vi "Get Sensor Objects Signals.vi"(7 "Filter Cluster":string="RDB_SENSOR_STATE", 8 "error in (no error)":errorcluster) -> (0 "error out (no error)":errorcluster, 1 "Sensor Signals":string[](array[string]), 2 "Sensor Names":string[](array[string]))   [LabVIEW 2023, in "Vires VTD System Explorer.lvlib"]
uses:
  Vires VTD System Explorer.lvlib
  <vilib>/xnet/xnet.llb/XNET String To IO Name (Database Alias).vi
  <resource>/objmgr/xnet.rc
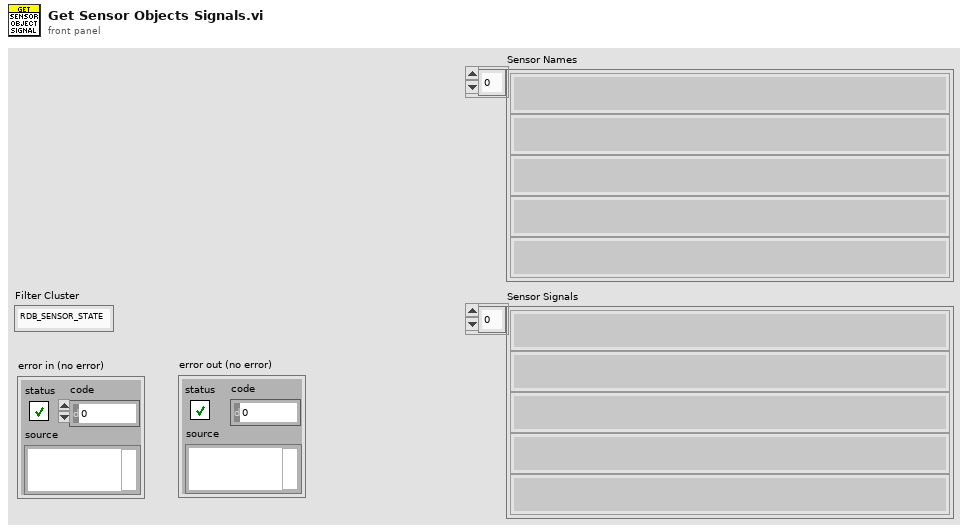
[diagram p1: front panel]
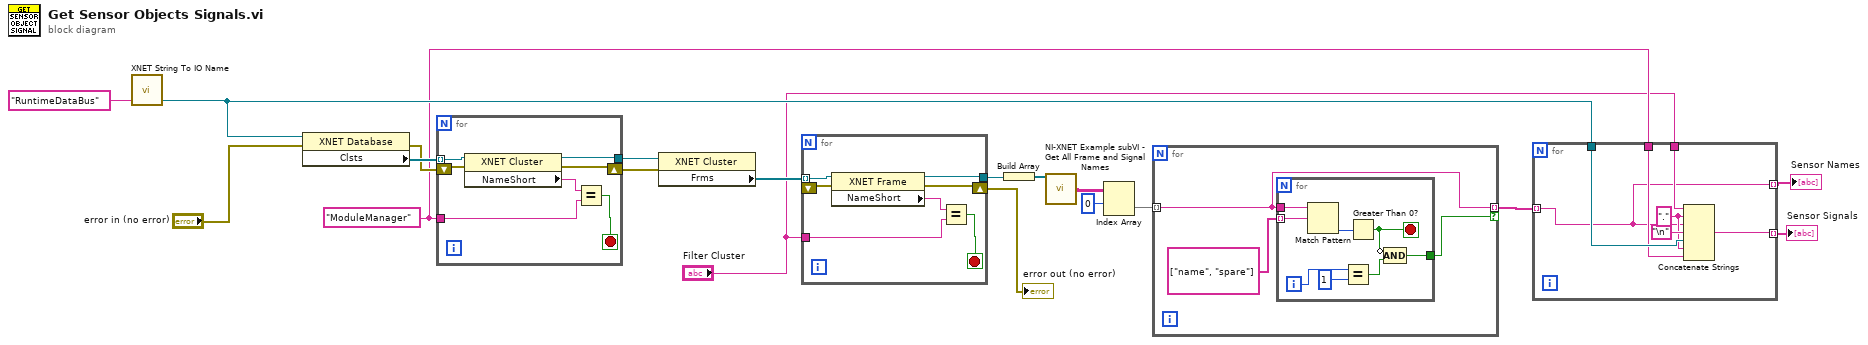
[diagram p0: block diagram]
diagram:
  w6 = "ModuleManager" ("Filter Cluster")
  n1 = call-poly <vilib>:"XNET String To IO Name.vi"("string"="RuntimeDataBus" ("element")) -> ("XNET Database"=w7:refnum<k21>)  [unwired: 4 out]
  n2 = property class="XNET Database"(reference=w7, error in="error in (no error)") -> (error out=w17:errorcluster, "Clsts"=w18:refnum<k21>[])  [unwired: 1 out]
  n3 = for {
    tunnel: w18 -> [w26] mode=indexing
    tunnel: [w25] -> w16
    shift-right: [w21] -> w15
    shift-left: w17 -> [w22]
    tunnel: w6 -> [w20]
    stop <- w24 stop-if-true
    n4 = property class="XNET Cluster"(reference=w26, error in=w22) -> (reference out=w25:refnum<k21>, error out=w21:errorcluster, "NameShort"=w23:string)
    n5 = Equal?(x=w23, y=w20) -> (x = y?=w24:bool)
  }
  n6 = property class="XNET Cluster"(reference=w16, error in=w15) -> ("Frms"=w14:refnum<k21>[])  [unwired: 2 out]
  n7 = for {
    tunnel: w14 -> [w33] mode=indexing
    tunnel: [w32] -> w13
    shift-right: [w28] -> w1
    shift-left: _ -> [w29]
    tunnel: "Filter Cluster" -> [w27]
    stop <- w31 stop-if-true
    n8 = property class="XNET Frame"(reference=w33, error in=w29) -> (reference out=w32:refnum<k21>, error out=w28:errorcluster, "NameShort"=w30:string)
    n9 = Equal?(x=w30, y=w27) -> (x = y?=w31:bool)
  }
  "error out (no error)" <- w1
  n10 = Build Array(w13) -> (w12:refnum<k21>[])
  n11 = call "NI-XNET Example subVI - Get All Frame and Signal Names.vi"("XNET Frames"=w12) -> ("Signal Names"=w10:string[][])  [unwired: 10 in, 4 out]
  n12 = Index Array(array=w10, index (row)=0) -> (element=w9:string[])  [unwired: 1 in]
  n13 = for {
    tunnel: w9 -> [w35] mode=indexing
    tunnel: [w35] -> w8 mode=indexing if=w34
    n14 = for {
      tunnel: string[] ["name", "spare"] -> [w44] mode=indexing
      tunnel: w35 -> [w43]
      tunnel: [w37] -> w34
      i -> [w42]
      stop <- w38 stop-if-true
      n15 = Match Pattern(string=w43, regular expression=w44) -> (offset past match=w40:i32)  [unwired: 1 in, 3 out]
      n16 = Equal?(x=w42, y=1) -> (x = y?=w39:bool)
      n17 = Greater Than 0?(x=w40) -> (x > 0?=w38:bool)
      n18 = Compound Arithmetic op=AND(invert w38, w39) -> (w37:bool)
    }
  }
  n19 = for {
    tunnel: w8 -> [w45] mode=indexing
    tunnel: "Filter Cluster" -> [w47]
    tunnel: w7 -> [w50]
    tunnel: w6 -> [w49]
    tunnel: [w48] -> w5 mode=indexing
    tunnel: [w45] -> w3 mode=indexing
    w46 = "." ("string")
    n20 = Concatenate Strings(w47, w46, w45, "\n", w50, w46, w49) -> (w48:string)
  }
  "Sensor Signals" <- w5
  "Sensor Names" <- w3
